vi "Main_Robot_Control.vi"() -> ()   [LabVIEW 2014]
uses:
  <vilib>/Platform/TimedLoop/XDataNode/timing_clust.ctl
  <vilib>/Platform/TimedLoop/XDataNode/nitl_modes.ctl
  <vilib>/Platform/TimedLoop/XDataNode/wakeup.ctl
  <vilib>/Platform/TimedLoop/XDataNode/XDataNode.xnode
  <vilib>/Platform/TimedLoop/XDataNode/XDNodeRunTimeDep.lvlib
panel:
  out "LIDAR Object Point":i32
  in  "Tab Control":T1(tab)
  out "Sharp IR Chart":dynamicdata(graph)
  in  "Motor Direction":bool
  out "Sharp IR":i16(slide) scale=0.0..5.0
  out "Potentiometer":i32(slide) scale=0.0..5.0
  out "Scaled Sharp IR Chart":dynamicdata(graph)
  out "LIDAR":bool
  out "Location":i32
  out "Width":i32
  out "Previous Iteration Finished Late?":bool
  in  "stop":bool
  # "E-STOP"
  # "See the block diagram for modification instructions."
  # "CCW"
  # "CCW"
  # "CW"
  # "LIDAR"
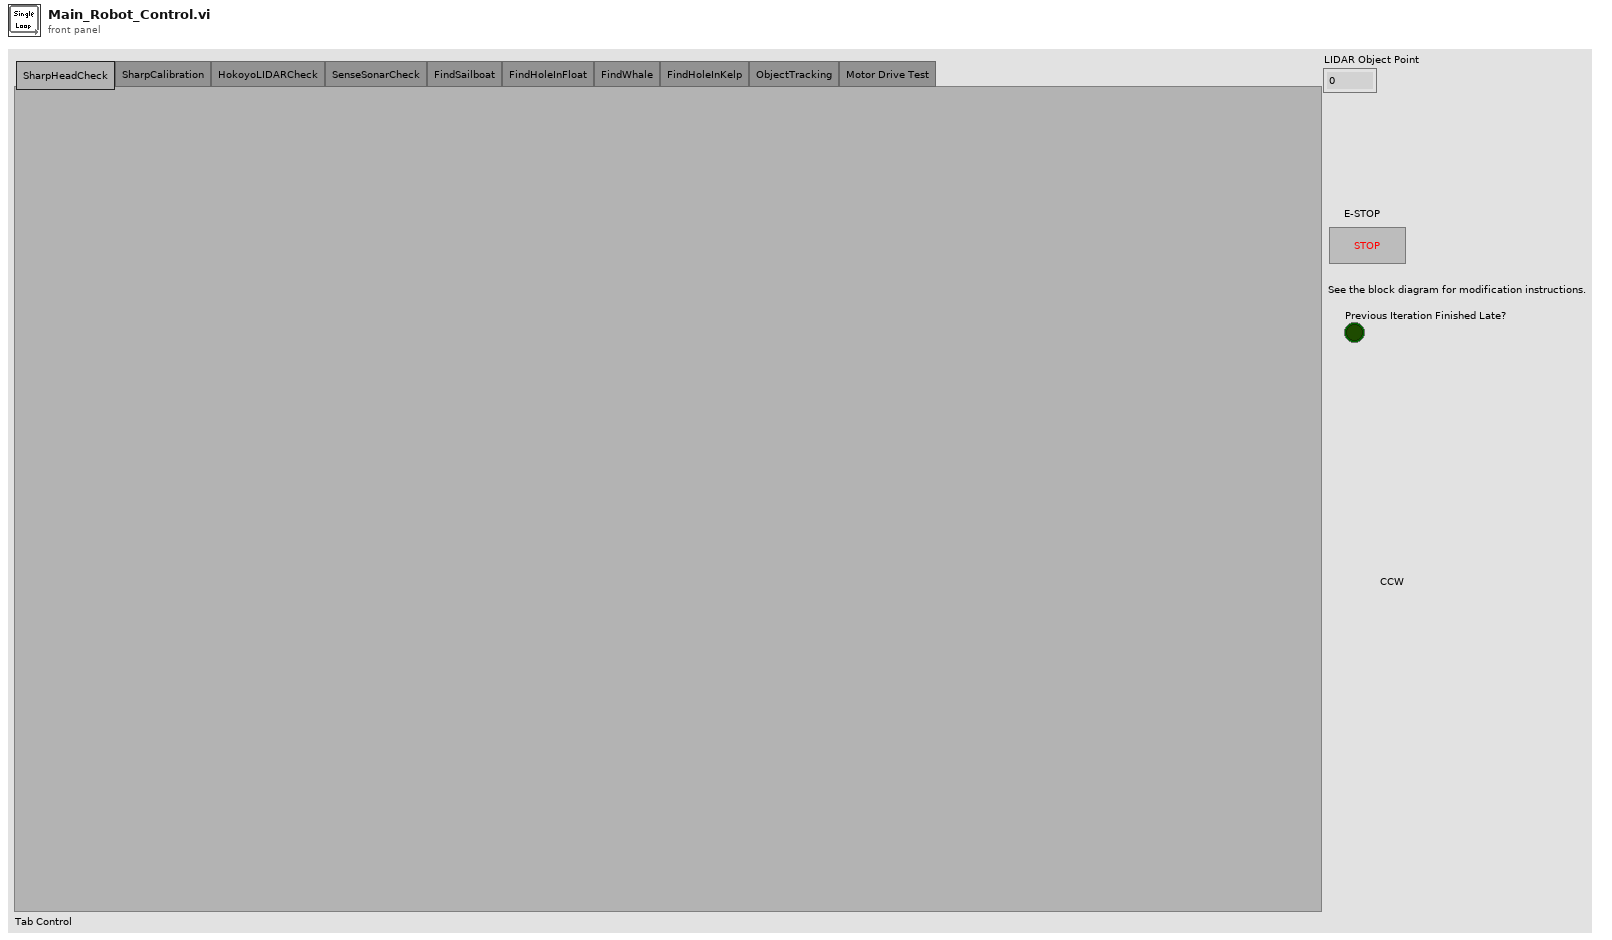
[diagram p1: front panel]
types:
  T1 = enum32{"SharpHeadCheck", "SharpCalibration", "HokoyoLIDARCheck", "SenseSonarCheck", "FindSailboat", "FindHoleInFloat", "FindWhale", "FindHoleInKelp", "ObjectTracking", "Motor Drive Test"}
  T2 = typedef "XDNodeRunTimeDep.lvlib/timing_clust.ctl" = cluster{"Expected End [f-1]":u64, "Actual End [f-1]":u64, "Finished Late? [f-1]":bool, "Expected End [i-1]":u64, "Actual End [i-1]":u64, "Finished Late? [i-1]":bool, "Expected Start [i]":u64, "Actual Start [i]":u64, "Expected Start [f]":u64, "Actual Start [f]":u64, "Source Name":string, "Structure Name":string, "Period":i64, "Deadline":i64, "Offset":i64, "Start":i64, "Priority":i32, "Timeout":i32, "Mode":T3, "Wakeup Reason":T4, "Error":errorcluster, "Source Type":string, "Secondary Source Type":string, "Global End Time":u64, "Global Start Time":u64, "Frame Duration":u64, "Iteration Duration":u64, "Assigned CPU":i32, "I/O Scan Engine Mode":u32}
  T3 = typedef "XDNodeRunTimeDep.lvlib/nitl_modes.ctl" = enum32{"No Change", "Process missed periods, maintain original phase", "Discard missed periods, maintain original phase", "Process missed periods, ignore original phase", "Discard missed periods, ignore original phase"}
  T4 = typedef "XDNodeRunTimeDep.lvlib/wakeup.ctl" = enum32{"Normal", "Aborted", "Asynchronous wakeup", "Timing source error", "Timed loop error", "Timeout"}
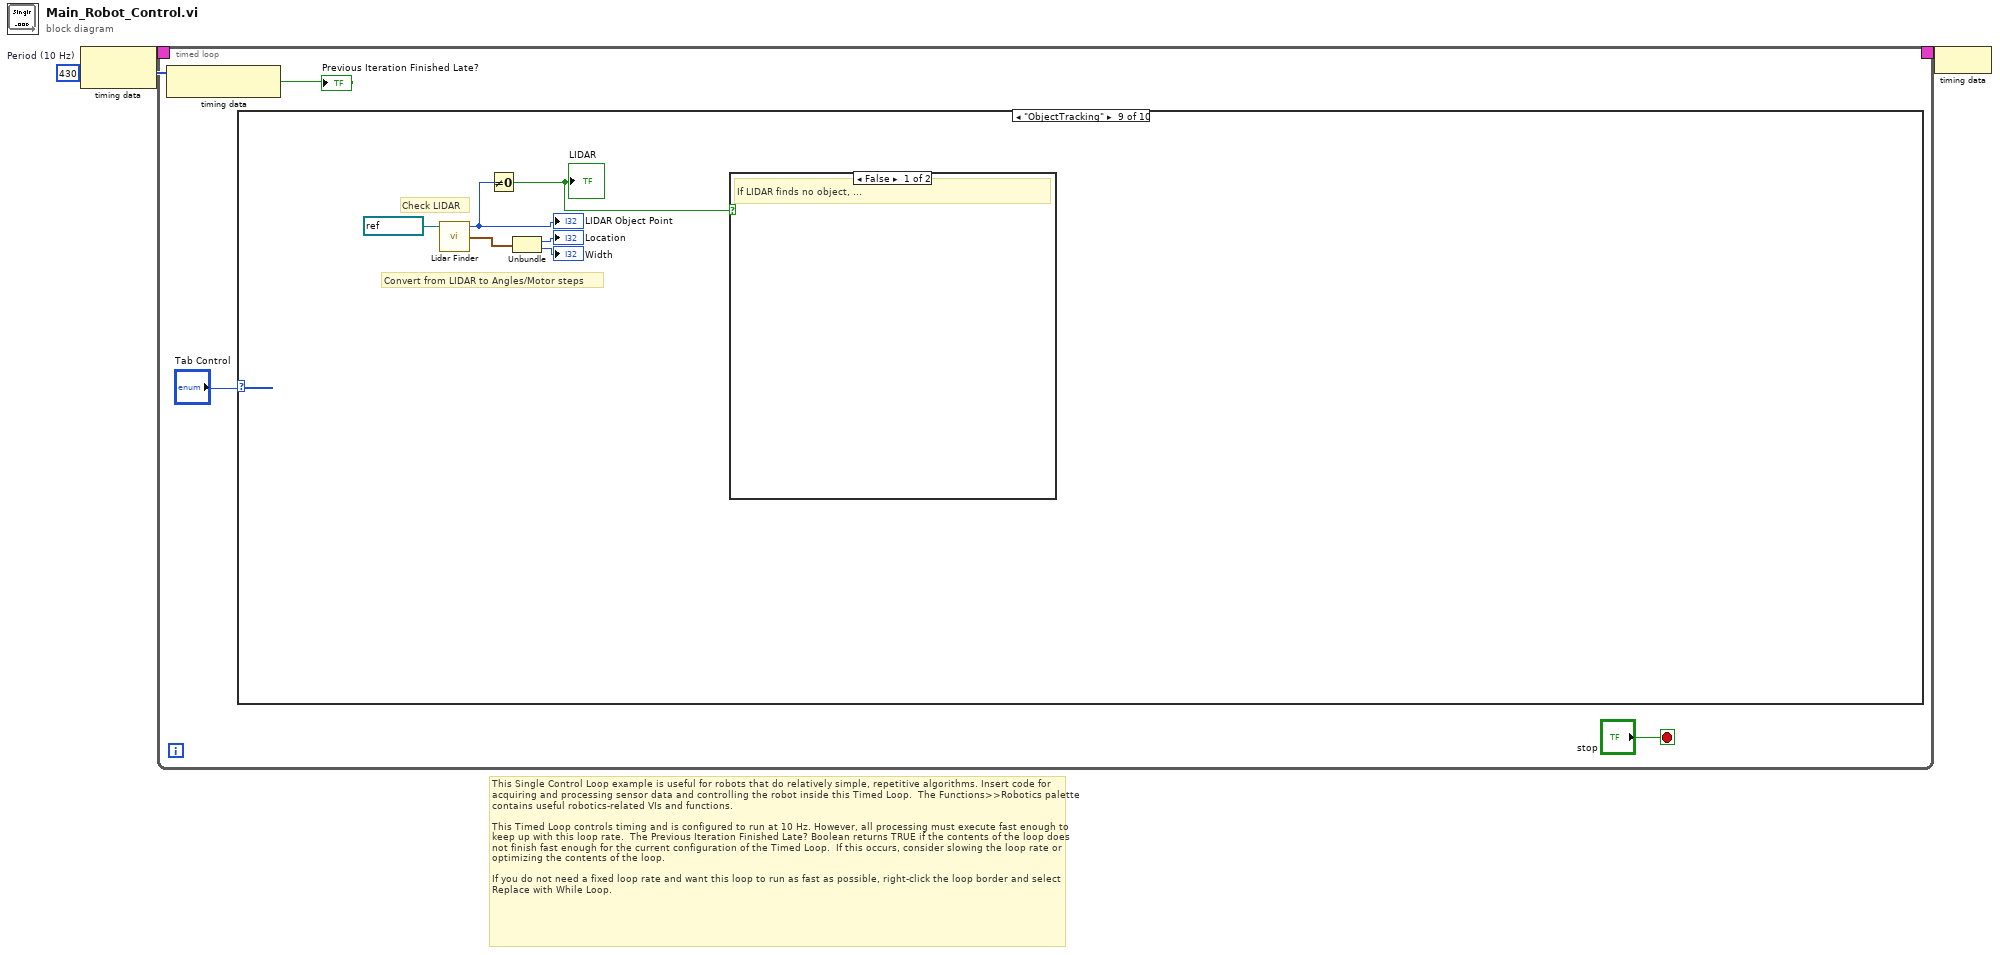
[diagram p0: block diagram]
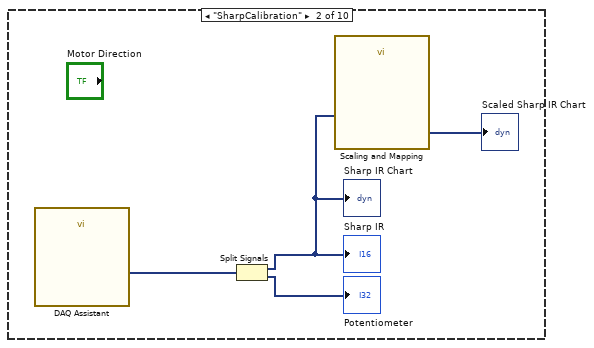
[diagram p3: hidden frame]
diagram:
  w1 = i64 430  # Period (10 Hz)
  # "This Single Control Loop example is useful for robots that do relatively simple, repetitive algorithms. Insert code for acquiring and processing sensor data and controlling the robot inside this Timed Loop.  The Functions>>Robotics palette contains useful robotics-related VIs and functions.\n\nThis Timed Loop controls timing and is configured to run at 10 Hz. However, all processing must execute fast enough to keep up with this loop rate.  The Previous Iteration Finished Late? Boolean returns TRUE if the contents of the loop does not finish fast enough for the current configuration of the Timed Loop.  If this occurs, consider slowing the loop rate or optimizing the contents of the loop.\n\nIf you do not need a fixed loop rate and want this loop to run as fast as possible, right-click the loop border and select Replace with While Loop."
  n1 = node-c288(w1) -> (w3:T2)
  n2 = timed-loop {
    timing: w3 -> [_]
    timing-out: [_] -> w2
    stop <- "stop" stop-if-true
    n3 = node-c288() -> (→"Previous Iteration Finished Late?":bool)  [unwired: 1 in]
    n4 = case shown="\"ObjectTracking\"" "Tab Control" {
      frame "SharpHeadCheck", Default {
      }
      frame "SharpCalibration" {
        n5 = call "DAQ Assistant"() -> ("data"=w10:dynamicdata)  [unwired: 17 in, 2 out]
        n6 = Split Signals(w10) -> (w8:dynamicdata, →"Potentiometer":dynamicdata)  [unwired: 2 in]
        "Sharp IR" <- w8
        "Sharp IR Chart" <- w8
        n7 = call "Scaling and Mapping"("Signals"=w8) -> ("Scaled Signals"=→"Scaled Sharp IR Chart":dynamicdata)  [unwired: 9 in, 1 out]
      }
      frame "HokoyoLIDARCheck" {
      }
      frame "SenseSonarCheck" {
      }
      frame "FindSailboat" {
      }
      frame "FindHoleInFloat" {
      }
      frame "FindWhale" {
      }
      frame "FindHoleInKelp" {
      }
      frame "ObjectTracking" {
        # "Convert from LIDAR to Angles/Motor steps"
        # "Check LIDAR"
        n8 = call "Lidar Finder.vi"("VISA resource name"=refnum<visa-resource-name> "COM4") -> ("Widest Object"=w15:cluster{i32, i32}, "Where to Point"=w12:i32)  [unwired: 2 in, 1 out]
        "LIDAR Object Point" <- w12
        n9 = Not Equal To 0?(x=w12) -> (x != 0?=w11:bool)
        "LIDAR" <- w11
        n10 = Unbundle(w15) -> (→"Location":i32, →"Width":i32)
        n11 = case shown="False" w11 {
          frame False {
            # "If LIDAR finds no object, ..."
          }
          frame True {
            # "If LIDAR has found an object, ..."
          }
        }
      }
      frame "Motor Drive Test" {
      }
    }
  }
  n12 = node-c288(w2) -> ()
